vi "save control values.vi"(5 "Append timestamp (true)":bool=TRUE, 6 "error in":errorcluster, 7 "Save only this":string[](array[string]), 8 "Dont save":string[](array[string]), 9 "Path":path) -> (0 "error out":errorcluster, 3 "file path out":path)   [LabVIEW 2020, in "POLARIS Vision utility.lvlib"]
doc: "from ni.com \nauthor mmiers."
uses:
  POLARIS Vision utility.lvlib
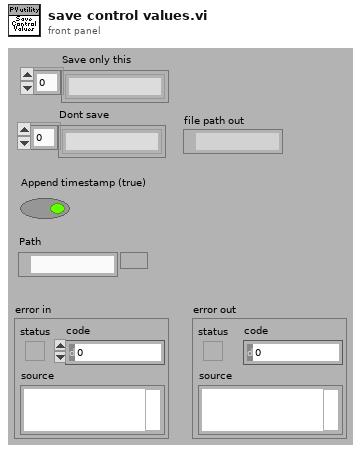
[diagram p1: front panel]
types:
  T1 = cluster{"Name":string, "type string":i16[], "data string":string}[]
  T2 = enum32{"invalid app kind", "Development System", "Run Time System", "Student Edition", "Embedded LabVIEW", "Evaluation", "Custom"}
  T3 = cluster{"Name":string, "type string":i16[], "data string":string}
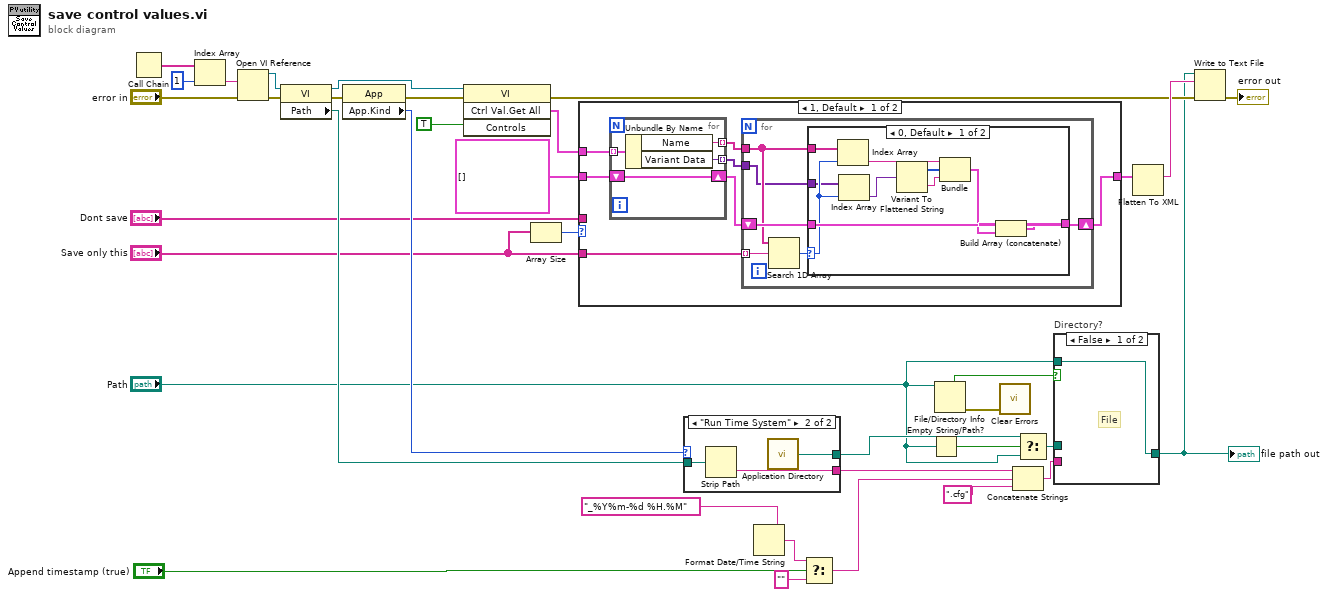
[diagram p0: block diagram]
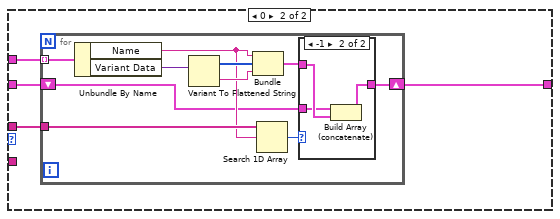
[diagram p3: hidden frame]
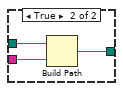
[diagram p5: hidden frame]
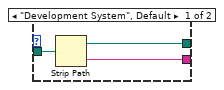
[diagram p6: hidden frame]
diagram:
  n1 = Call Chain() -> (call chain=w31:string[])
  n2 = Index Array(array=w31, index=1) -> (element=w27:string)
  n3 = Open VI Reference(vi path=w27, error in (no error)="error in") -> (vi reference=w26:refnum<vi>, error out=w28:errorcluster)  [unwired: 4 in]
  n4 = property class="VI"(reference=w26, error in=w28) -> (reference out=w6:refnum<vi>, error out=w23:errorcluster, "Path"=w25:path)
  n5 = property class="App"(error in=w23) -> (error out=w22:errorcluster, "App.Kind"=w24:T2)  [unwired: 1 in, 1 out]
  n6 = invoke class="VI" method="Ctrl Val.Get All"(reference=w6, error in=w22, "Controls"=TRUE ("Save control values")) -> (error out=w33:errorcluster, "Get All Control Values Variant"=w4:cluster{"Name":string, "Variant Data":variant}[])  [unwired: 1 in, 2 out]
  n7 = Array Size(array="Save only this") -> (size(s)=w2:i32)
  n8 = case shown="1, Default" w2 {
    tunnel: [w37 w68] -> w34
    tunnel: "Dont save" -> [_ w67]
    tunnel: w4 -> [w43 w66]
    tunnel: T1 [] -> [w42 w65]
    tunnel: "Save only this" -> [w39 _]
    frame 1, Default {
      n9 = for {
        tunnel: w43 -> [w64] mode=indexing
        shift-right: [w63] -> w38
        shift-left: w42 -> [w63]
        tunnel: [w62] -> w40 mode=indexing
        tunnel: [w61] -> w41 mode=indexing
        n10 = Unbundle By Name(w64) -> ("Name"=w61:string, "Variant Data"=w62:variant)
      }
      n11 = for {
        tunnel: w41 -> [w45]
        tunnel: w40 -> [w44]
        tunnel: w39 -> [w48] mode=indexing
        shift-right: [w46] -> w37
        shift-left: w38 -> [w47]
        n12 = Search 1D Array(1D array=w45, element=w48) -> (index of element=w49:i32)  [unwired: 1 in]
        n13 = case shown="0, Default" w49 {
          selector: w49 -> [w53 _]
          tunnel: [w59 w60] -> w46
          tunnel: w47 -> [w58 w60]
          tunnel: w45 -> [w54 _]
          tunnel: w44 -> [w52 _]
          frame 0, Default {
            n14 = Index Array(array=w54, index=w53) -> (element=w55:string)
            n15 = Index Array(array=w52, index=w53) -> (element=w51:variant)
            n16 = Variant To Flattened String(Variant=w51) -> (data string=w56:string, 1:w57:i16[])
            n17 = Bundle("Name"=w55, "type string"=w57, "data string"=w56) -> (w50:T3)  [unwired: 1 out]
            n18 = Build Array (concatenate)(w58, w50) -> (w59:T1)
          }
          frame -1 {
          }
        }
      }
    }
    frame 0 {
      n19 = for {
        tunnel: w66 -> [w75] mode=indexing
        tunnel: w67 -> [w74]
        shift-right: [w70] -> w68
        shift-left: w65 -> [w69]
        n20 = Unbundle By Name(w75) -> ("Name"=w73:string, "Variant Data"=w78:variant)
        n21 = Variant To Flattened String(Variant=w78) -> (data string=w76:string, 1:w77:i16[])
        n22 = Bundle("Name"=w73, "type string"=w77, "data string"=w76) -> (w71:T3)  [unwired: 1 out]
        n23 = Search 1D Array(1D array=w74, element=w73) -> (index of element=w72:i32)  [unwired: 1 in]
        n24 = case shown="-1" w72 {
          tunnel: w71 -> [_ w82]
          tunnel: [w79 w81] -> w70
          tunnel: w69 -> [w79 w80]
          frame 0, Default {
          }
          frame -1 {
            n25 = Build Array (concatenate)(w80, w82) -> (w81:T1)
          }
        }
      }
    }
  }
  n26 = case shown="\"Run Time System\"" w24 {
    tunnel: w25 -> [w85 w88]
    tunnel: [w84 w87] -> w12
    tunnel: [w83 w86] -> w17
    frame "Development System", Default {
      n27 = Strip Path(path=w85) -> (stripped path=w84:path, name=w83:string)
    }
    frame "Run Time System" {
      n28 = Strip Path(path=w88) -> (name=w86:string)  [unwired: 1 out]
      n29 = call <vilib>:"Application Directory.vi"() -> ("Application Directory"=w87:path)
    }
  }
  n30 = Format Date/Time String(time format string (%c)="_%Y%m-%d %H.%M") -> (date/time string=w15:string)  [unwired: 2 in]
  n31 = Select(t=w15, s="Append timestamp (true)", f="") -> (s? t:f=w14:string)
  n32 = Empty String/Path?(string/path="Path") -> (empty?=w11:bool)
  n33 = File/Directory Info(path="Path") -> (directory=w9:bool, error out=w7:errorcluster)  [unwired: 1 in, 5 out]
  n34 = call <vilib>:"Clear Errors.vi"("error in (no error)"=w7) -> ()  [unwired: 5 in, 2 out]
  n35 = Concatenate Strings(w17, w14, ".cfg" ("string")) -> (w20:string)
  n36 = Select(t=w12, s=w11, f="Path") -> (s? t:f=w10:path)
  n37 = case "Directory?" shown="False" w9 {
    tunnel: [w89 w92] -> w21
    tunnel: w20 -> [_ w91]
    tunnel: w10 -> [_ w90]
    tunnel: "Path" -> [w89 _]
    frame False {
      # "File"
    }
    frame True {
      n38 = Build Path(base path=w90, name or relative path=w91) -> (appended path=w92:path)
    }
  }
  "file path out" <- w21
  n39 = Flatten To XML(6:w34) -> (2:w35:string)
  n40 = Write to Text File(file (use dialog)=w21, text=w35, error in=w33) -> (error out=→"error out":errorcluster)  [unwired: 3 out]
